vi "Read Died Broadcast.vi"(11 "JQMHStartup in":refnum<class "RQMHStartup.lvclass">) -> (2 "Died Broadcast":refnum<user-event>, 3 "JQMHStartup out":refnum<class "RQMHStartup.lvclass">)   [LabVIEW 2024, in "RQMHStartup.lvclass"]
uses:
  RQMHStartup.lvclass
  Shared/Died.ctl
  RQMHStartup.lvclass/RQMHStartup.ctl
  Shared/JQMHShared.lvlib
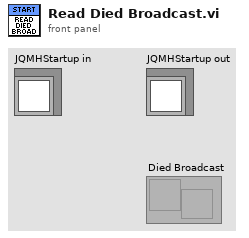
[diagram p1: front panel]
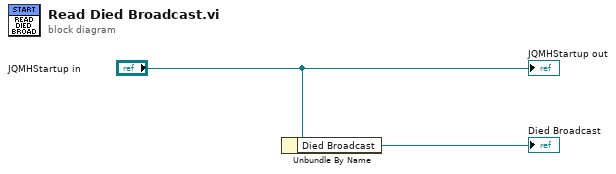
[diagram p0: block diagram]
diagram:
  n1 = Unbundle By Name("JQMHStartup in") -> ("Died Broadcast"=→"Died Broadcast":refnum<user-event>)
  "JQMHStartup out" <- "JQMHStartup in"
